vi "Set Light HSB By ID.vi"(7 "ID":u8, 8 "Error In":errorcluster, 10 "HSB":T1={"Hue"=0, "Saturation"=255, "Brightness"=255}, 11 "Hue Config":T2) -> (0 "Error Out":errorcluster, 3 "Hue Config":T2)   [LabVIEW 2013, in "LMH-Hue.lvlib"]
uses:
  LMH-Hue.lvlib
  Type Defs/Hue Ref.ctl
  <vilib>/httpClient/ClientHandle.ctl
  Type Defs/Light.ctl
  Type Defs/HSB.ctl
  Type Defs/JSON/Hue Sat Bri.ctl
  <vilib>/httpClient/PUTBuffer.vi
  <vilib>/httpClient/LabVIEWHTTPClient.lvlib
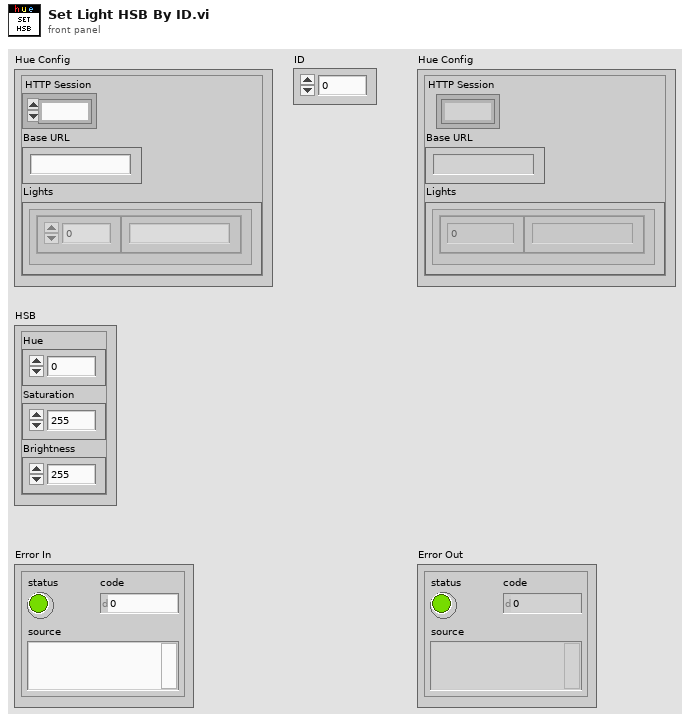
[diagram p1: front panel]
types:
  T1 = typedef "LMH-Hue.lvlib/HSB.ctl" = cluster{"Hue":u16, "Saturation":u8, "Brightness":u8}
  T2 = typedef "LMH-Hue.lvlib/Hue Ref.ctl" = cluster{"HTTP Session":T3, "Base URL":string, "Lights":T4[]}
  T3 = typedef "LabVIEWHTTPClient.lvlib/ClientHandle.ctl" = refnum<k1>
  T4 = typedef "LMH-Hue.lvlib/Light.ctl" = cluster{"ID":i32, "Name":string}
  T5 = typedef "LMH-Hue.lvlib/Hue Sat Bri.ctl" = cluster{"hue":u16, "sat":u8, "bri":u8}
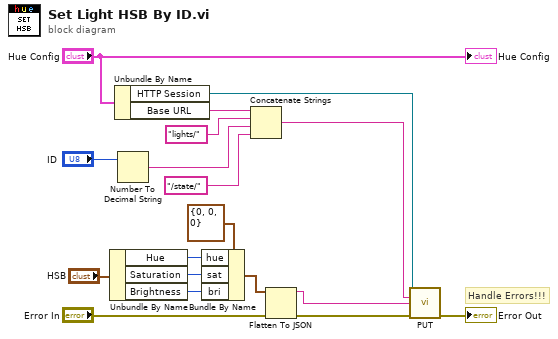
[diagram p0: block diagram]
diagram:
  # "Handle Errors!!!"
  n1 = Unbundle By Name("HSB") -> ("Hue"=w4:u16, "Saturation"=w2:u8, "Brightness"=w3:u8)
  n2 = Unbundle By Name("Hue Config") -> ("HTTP Session"=w17:T3, "Base URL"=w7:string)
  n3 = Number To Decimal String(number="ID") -> (decimal integer string=w9:string)  [unwired: 1 in]
  n4 = Bundle By Name(cluster=T5 {"hue"=0, "sat"=0, "bri"=0} ("Hue Sat Bri"), "hue"=w4, "sat"=w2, "bri"=w3) -> (w16:T5)
  n5 = Concatenate Strings(w7, "lights/" ("string"), w9, "/state/" ("string")) -> (w13:string)
  n6 = Flatten To JSON(anything=w16, error in (no error)="Error In") -> (JSON string=w5:string, 11:w12:errorcluster)  [unwired: 1 in]
  n7 = call-poly <vilib>:"PUT.vi"("client handle"=w17, "url"=w13, "buffer"=w5, "error in (no error)"=w12) -> ("error out"=→"Error Out":errorcluster)  [unwired: 8 in, 3 out]
  "Hue Config" <- "Hue Config"
